vi "GlobalParcelLocker.vi"() -> ()   [LabVIEW 2017]
panel:
  out "Parcel locker":u32
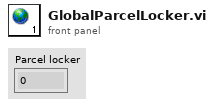
[diagram p1: front panel]
diagram:
